vi "Camera Control.vi"(9 "Y Degrees":dbl, 11 "X  Degrees":dbl) -> ()   [LabVIEW 2013]
uses:
  Robot Global Data.vi
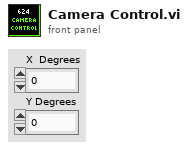
[diagram p1: front panel]
types:
  T1 = typedef "WPI_ServoDeviceRef.ctl" = cluster{"DeviceStatus":errorcluster, "Digital Module":T2, "PWM Channel":T3, "DeadBand":T4}
  T2 = typedef "FPGA_TypedefDigitalModule.ctl" = enum16{"Digital Module 1", "Digital Module 2"}
  T3 = typedef "FPGA_DIOPWMChannel.ctl" = enum8{"PWM 1", "PWM 2", "PWM 3", "PWM 4", "PWM 5", "PWM 6", "PWM 7", "PWM 8", "PWM 9", "PWM 10", "Invalid"}
  T4 = typedef "WPI_PWMDeadband.ctl" = cluster{"Name":string, "maxPositivePwm":i32, "minPositivePwm":i32, "centerPwm":i32, "maxNegativePwm":i32, "minNegativePwm":i32, "angularRange":u16}
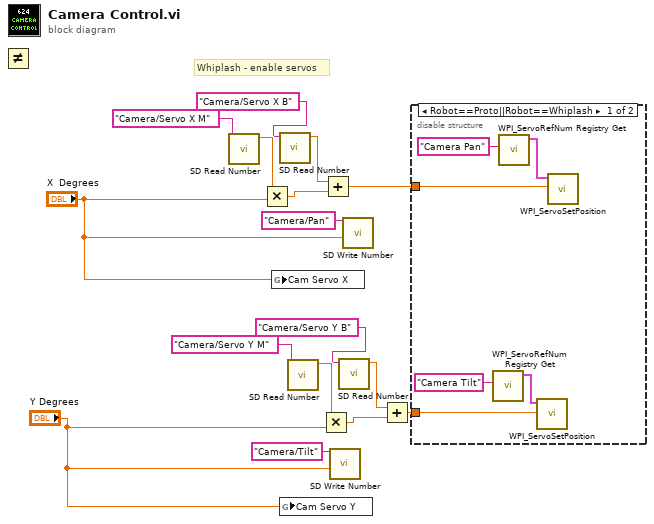
[diagram p0: block diagram]
diagram:
  # "Whiplash - enable servos"
  n1 = Not Equal?() -> ()  [unwired: 2 in, 1 out]
  n2 = call <vilib>:"SD Read Number.vi"("Name"="Camera/Servo X M") -> ("Numeric"=w13:dbl)  [unwired: 8 in, 2 out]
  n3 = Multiply(x=w13, y="X  Degrees") -> (x*y=w14:dbl)
  n4 = global write "Robot Global Data.vi" "Cam Servo X"("X  Degrees") -> ()
  n5 = call <vilib>:"SD Read Number.vi"("Name"="Camera/Servo X B") -> ("Numeric"=w10:dbl)  [unwired: 8 in, 2 out]
  n6 = global write "Robot Global Data.vi" "Cam Servo Y"("Y Degrees") -> ()
  n7 = call <vilib>:"SD Read Number.vi"("Name"="Camera/Servo Y M") -> ("Numeric"=w5:dbl)  [unwired: 8 in, 2 out]
  n8 = Multiply(x=w5, y="Y Degrees") -> (x*y=w6:dbl)
  n9 = Add(x=w10, y=w14) -> (x+y=w11:dbl)
  n10 = call <vilib>:"SD Write Number.vi"("Numeric"="Y Degrees", "Name"="Camera/Tilt") -> ()  [unwired: 8 in, 2 out]
  n11 = call <vilib>:"SD Read Number.vi"("Name"="Camera/Servo Y B") -> ("Numeric"=w2:dbl)  [unwired: 8 in, 2 out]
  n12 = call <vilib>:"SD Write Number.vi"("Numeric"="X  Degrees", "Name"="Camera/Pan") -> ()  [unwired: 8 in, 2 out]
  n13 = Add(x=w2, y=w6) -> (x+y=w3:dbl)
  n14 = disable-structure shown="Robot==Proto||Robot==Whiplash" {
    disable-tunnel: w11 -> [w22 _]
    disable-tunnel: w3 -> [w19 _]
    frame condition #0 (active) {
      n15 = call <vilib>:"WPI_ServoRefNum Registry Get.vi"("refnum name"="Camera Tilt") -> ("ServoDeviceRef"=w18:T1)  [unwired: 9 in, 1 out]
      n16 = call <vilib>:"WPI_ServoRefNum Registry Get.vi"("refnum name"="Camera Pan") -> ("ServoDeviceRef"=w21:T1)  [unwired: 9 in, 1 out]
      n17 = call <vilib>:"WPI_ServoSetPosition.vi"("Position"=w19, "ServoDeviceRef"=w18) -> ()  [unwired: 8 in, 2 out]
      n18 = call <vilib>:"WPI_ServoSetPosition.vi"("Position"=w22, "ServoDeviceRef"=w21) -> ()  [unwired: 8 in, 2 out]
    }
    frame condition #1 {
    }
  }
